vi "010 Gràfic XY.vi"() -> ()   [LabVIEW 2019]
panel:
  in  "Array 2":dbl[](array[numeric])
  in  "Array":dbl[](array[numeric])
  out "XY Graph":cluster{"Array":dbl[], "Array 2":dbl[]}(graph)
  in  "stop":bool
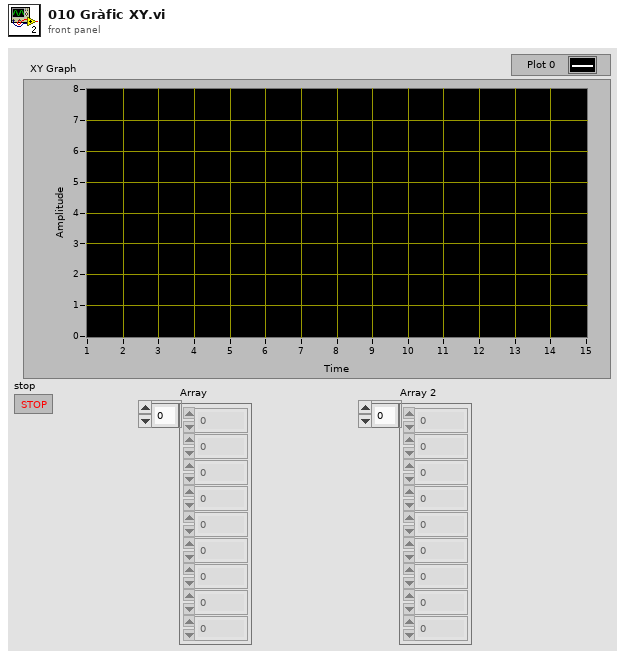
[diagram p1: front panel]
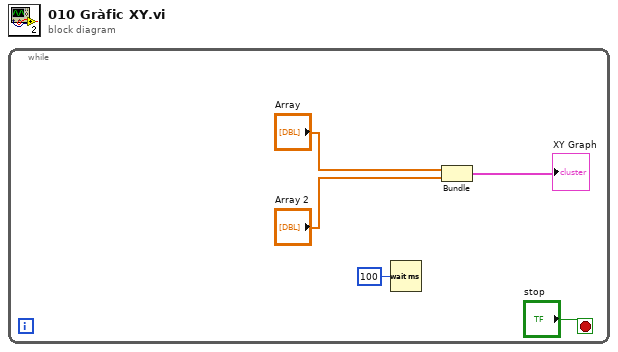
[diagram p0: block diagram]
diagram:
  n1 = while {
    stop <- "stop" stop-if-true
    n2 = Wait (ms)(milliseconds to wait=u32 100) -> ()  [unwired: 1 out]
    n3 = Bundle("Array"="Array", "Array 2"="Array 2") -> (→"XY Graph":cluster{"Array":dbl[], "Array 2":dbl[]})  [unwired: 1 in]
  }
